vi "DCMotor.vi"(6 "INB":bool, 7 "PWM":u16(ring) items=["PWM1", "PWM2", "PWM3", "PWM4"], 8 "error in (no error)":errorcluster, 9 "INA":bool, 10 "Duty Cycle":dbl min=0.0 max=255.0 step=1.0, 11 "CAN in":refnum<class "CAN.lvclass">) -> (0 "error out":errorcluster, 3 "CAN out":refnum<class "CAN.lvclass">)   [LabVIEW 2020]
uses:
  <vilib>/High Genius/HG_WSI_Tookit/Dependencies/Library/CAN/CAN.lvclass
  C:/Program Files (x86)/National Instruments/LabVIEW 2020/vi.lib/High Genius/HG_WSI_Tookit/Dependencies/Library/HG_LIB/HG_LIB.lvclass
  <vilib>/High Genius/HG_WSI_Tookit/Dependencies/Library/HG_LIB/HG_LIB.lvclass
  <vilib>/High Genius/HG_WSI_Tookit/Dependencies/Library/VMX Library.lvlib
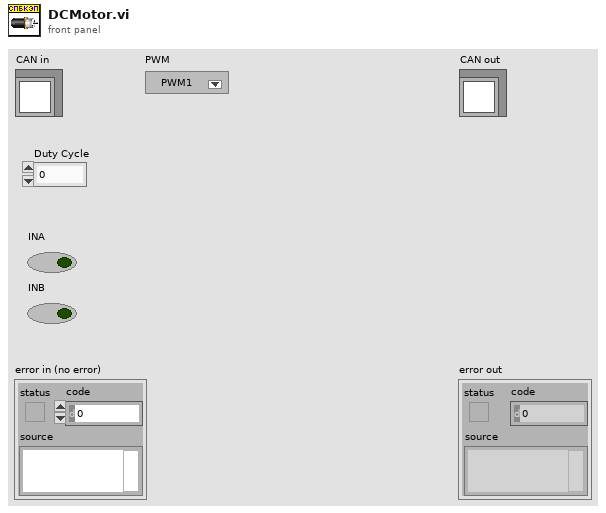
[diagram p1: front panel]
types:
  T1 = typedef "Semaphore RefNum" = refnum<k1>
  T2 = cluster{"titanenc0":i32, "titanenc1":i32, "titanenc2":i32, "titanenc3":i32, "rpm0":i16, "rpm1":i16, "rpm2":i16, "rpm3":i16, "resetenc0":bool, "resetenc1":bool, "resetenc2":bool, "resetenc3":bool}
  T3 = cluster{"data":cluster{"ai22":sgl, "ai23":sgl, "ai24":sgl, "ai25":sgl, "pulse12":i32, "pulse13":i32, "pwm14":i32, "pwm15":i32, "pwm16":dbl, "do17":bool, "do18":bool, "do19":bool, "do20":bool, "do21":bool, "di11":bool, "di9":bool, "motor0":u8, "motor1":u8, "motor2":u8, "motor3":u8, "dir00":u8, "dir01":u8, "dir02":u8, "dir03":u8, "dir10":u8, "dir11":u8, "dir12":u8, "dir13":u8, "limit0":bool, "limit1":bool, "limit2":bool, "limit3":bool, "limit4":bool, "limit5":bool, "limit6":bool, "limit7":bool, "lsb0H":u8, "lsb1H":u8, "lsb2H":u8, "lsb3H":u8, "lsb0L":u8, "lsb1L":u8, "lsb2L":u8, "lsb3L":u8, "enc0_counters":u32, "enc1_counters":u32, "enc2_counters":u32, "enc3_counters":u32, "counter10":u32, "counter8":u32, "reset_enc0":bool, "reset_enc1":bool, "reset_enc2":bool, "reset_enc3":bool, "pitch":sgl, "roll":sgl, "yaw":sgl, "zero_yaw":bool}}
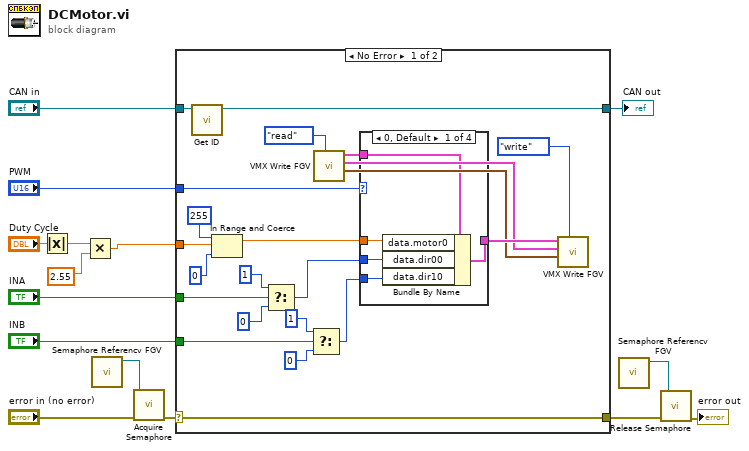
[diagram p0: block diagram]
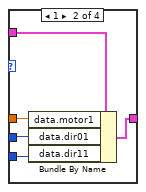
[diagram p2: hidden frame]
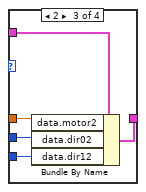
[diagram p3: hidden frame]
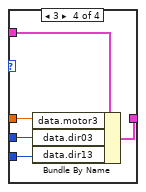
[diagram p4: hidden frame]
diagram:
  n1 = Absolute Value(x="Duty Cycle") -> (abs(x)=w8:dbl)
  n2 = Multiply(x=w8, y=2.55) -> (x*y=w1:dbl)
  n3 = call <vilib>:"Semaphore Referencv FGV.vi"() -> ("Semaphore Reference"=w3:T1)  [unwired: 11 in]
  n4 = call <vilib>:"Acquire Semaphore.vi"("error in (no error)"="error in (no error)", "semaphore"=w3) -> ("error out"=w7:errorcluster)  [unwired: 3 in, 2 out]
  n5 = case shown="No Error" w7 {
    selector: w7 -> [w25 w59]
    tunnel: [w25 w59] -> w5
    tunnel: [w37 w58] -> w14
    tunnel: "CAN in" -> [w36 w58]
    tunnel: "PWM" -> [w31 _]
    tunnel: "INB" -> [w28 _]
    tunnel: "INA" -> [w29 _]
    tunnel: w1 -> [w35 _]
    frame No Error {
      n6 = call <vilib>:"Get ID.vi"("HG_LIB in"=w36) -> ("HG_LIB out"=w37:refnum<class "CAN.lvclass">)  [unwired: 9 in, 1 out]
      n7 = In Range and Coerce(upper limit=255, x=w35, lower limit=0) -> (coerced(x)=w30:dbl)  [unwired: 1 out]
      n8 = Select(t=u8 1, s=w29, f=u8 0) -> (s? t:f=w27:u8)
      n9 = Select(t=u8 1, s=w28, f=u8 0) -> (s? t:f=w26:u8)
      n10 = call <vilib>:"VMX Write FGV.vi"("Enum"=enum16{"read", "write"}."read") -> ("Read Data3"=w20:cluster{"pwm17":i32, "pwm18":i32}, "Read Data2"=w21:T2, "Read Data"=w23:T3)  [unwired: 8 in]
      n11 = case shown="0, Default" w31 {
        tunnel: [w39 w47 w49 w54] -> w22
        tunnel: w30 -> [w42 w46 w52 w57]
        tunnel: w27 -> [w41 w45 w51 w56]
        tunnel: w26 -> [w40 w44 w50 w55]
        tunnel: w23 -> [w38 w43 w48 w53]
        frame 0, Default {
          n12 = Bundle By Name(cluster=w38, "data.motor0"=w42, "data.dir00"=w41, "data.dir10"=w40) -> (w39:T3)
        }
        frame 1 {
          n13 = Bundle By Name(cluster=w43, "data.motor1"=w46, "data.dir01"=w45, "data.dir11"=w44) -> (w47:T3)
        }
        frame 2 {
          n14 = Bundle By Name(cluster=w48, "data.motor2"=w52, "data.dir02"=w51, "data.dir12"=w50) -> (w49:T3)
        }
        frame 3 {
          n15 = Bundle By Name(cluster=w53, "data.motor3"=w57, "data.dir03"=w56, "data.dir13"=w55) -> (w54:T3)
        }
      }
      n16 = call <vilib>:"VMX Write FGV.vi"("Enum"=enum16{"read", "write"}."write", "Write Data3"=w20, "Write Data2"=w21, "Write Data"=w22) -> ()  [unwired: 5 in, 3 out]
    }
    frame Error {
    }
  }
  "CAN out" <- w14
  n17 = call <vilib>:"Semaphore Referencv FGV.vi"() -> ("Semaphore Reference"=w2:T1)  [unwired: 11 in]
  n18 = call <vilib>:"Release Semaphore.vi"("error in (no error)"=w5, "semaphore"=w2) -> ("error out"=→"error out":errorcluster)  [unwired: 4 in, 1 out]
